vi "OpGlobalSet.vi"(0 "ReloadButton":bool, 1 "Manuall servo":bool, 2 "Auton drag":bool, 5 "ThrowButton":bool, 7 "LobButton":bool, 9 "GrabButton":bool, 11 "GroundPassButton":bool, 12 "Shoulder joint":bool, 13 "Shoulder joint up":bool) -> ()   [LabVIEW 2014]
uses:
  Events.vi
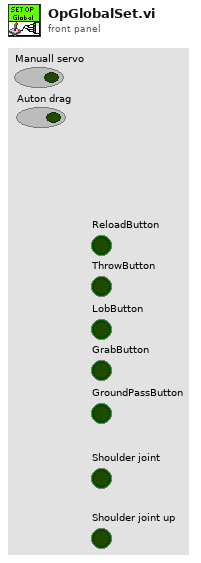
[diagram p1: front panel]
types:
  T1 = typedef "Eventgrab.ctl" = cluster{"Grab":bool, "GroundPass":bool, "Test Aqaure":dbl, "Shoulder up or down?":bool, "Auton drag":bool}
  T2 = cluster{"Reloading?":bool, "Throw":bool, "Ready?":bool, "Truss throw":bool, "Power is high?":bool, "Automatic relaod?":bool, "Manuall servo":bool}
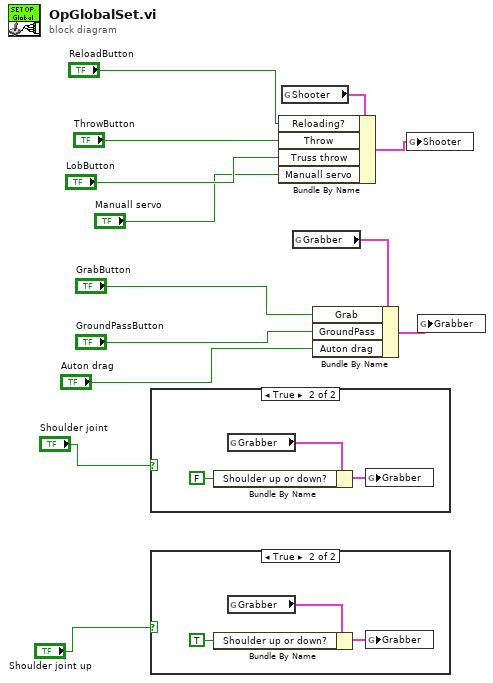
[diagram p0: block diagram]
diagram:
  n1 = case shown="True" "Shoulder joint" {
    frame False {
    }
    frame True {
      n2 = global read "Events.vi" "Grabber"() -> (w16:T1)
      n3 = Bundle By Name(cluster=w16, "Shoulder up or down?"=FALSE) -> (w15:T1)
      n4 = global write "Events.vi" "Grabber"(w15) -> ()
    }
  }
  n5 = case shown="True" "Shoulder joint up" {
    frame False {
    }
    frame True {
      n6 = global read "Events.vi" "Grabber"() -> (w19:T1)
      n7 = Bundle By Name(cluster=w19, "Shoulder up or down?"=TRUE) -> (w18:T1)
      n8 = global write "Events.vi" "Grabber"(w18) -> ()
    }
  }
  n9 = global read "Events.vi" "Shooter"() -> (w13:T2)
  n10 = Bundle By Name(cluster=w13, "Reloading?"="ReloadButton", "Throw"="ThrowButton", "Truss throw"="LobButton", "Manuall servo"="Manuall servo") -> (w11:T2)
  n11 = global read "Events.vi" "Grabber"() -> (w9:T1)
  n12 = Bundle By Name(cluster=w9, "Grab"="GrabButton", "GroundPass"="GroundPassButton", "Auton drag"="Auton drag") -> (w8:T1)
  n13 = global write "Events.vi" "Shooter"(w11) -> ()
  n14 = global write "Events.vi" "Grabber"(w8) -> ()
